vi "Camera routines.vi"   [LabVIEW 2017]
types:
  T1 = typedef "WPI_CameraDevRef.ctl" = cluster{"Camera Address":string, "CameraStatus":errorcluster}
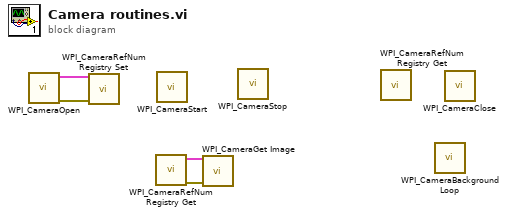
[diagram p0: block diagram]
diagram:
  n1 = call <vilib>:"WPI_CameraOpen.vi"() -> ("error out"=w4:errorcluster, "CameraDevRef"=w3:T1)  [unwired: 10 in]
  n2 = call <vilib>:"WPI_CameraRefNum Registry Set.vi"("error in (no error)"=w4, "CameraDevRef"=w3) -> ()  [unwired: 8 in, 2 out]
  n3 = call <vilib>:"WPI_CameraRefNum Registry Get.vi"() -> ("error out"=w2:errorcluster, "CameraDevRef"=w1:T1)  [unwired: 10 in]
  n4 = call <vilib>:"WPI_CameraStart.vi"() -> ()  [unwired: 10 in, 2 out]
  n5 = call <vilib>:"WPI_CameraGet Image.vi"("error in (no error)"=w2, "CameraDevRef"=w1) -> ()  [unwired: 7 in, 3 out]
  n6 = call <vilib>:"WPI_CameraStop.vi"() -> ()  [unwired: 10 in, 2 out]
  n7 = call <vilib>:"WPI_CameraRefNum Registry Get.vi"() -> ()  [unwired: 10 in, 2 out]
  n8 = call <vilib>:"WPI_CameraBackground Loop.vi"() -> ()  [unwired: 12 in]
  n9 = call <vilib>:"WPI_CameraClose.vi"() -> ()  [unwired: 11 in, 1 out]
